vi "Get Path Regex.vi"(8 "error in (no error)":errorcluster, 11 "TestAuthController in":refnum<class "TestAuthController.lvclass">) -> (0 "error out":errorcluster, 2 "Path Regex":string, 3 "TestAuthController out":refnum<class "TestAuthController.lvclass">)   [LabVIEW 2020, in "TestAuthController.lvclass"]
uses:
  TestAuthController.lvclass
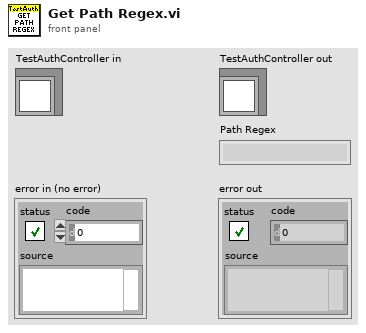
[diagram p1: front panel]
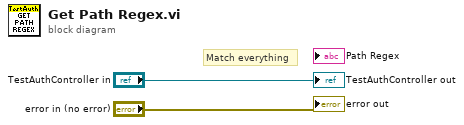
[diagram p0: block diagram]
diagram:
  # "Match everything"
  "error out" <- "error in (no error)"
  "TestAuthController out" <- "TestAuthController in"
